vi "FFT Testing.vi"() -> ()   [LabVIEW 2019]
uses:
  <vilib>/express/express analysis/Spectral/Block/exnSpectralBlock spectral measurements peak poly.vi
  <vilib>/express/express analysis/Spectral/Block/exnSpectralBlock spectral measurements peak DDT.vi
  <vilib>/express/express analysis/Spectral/XNode/ExpressSpectralMeasurementsBlockNode.xnode
panel:
  out "Freq Max":dbl
  out "Amp":dbl
  out "data":dynamicdata(graph)
  out "Waveform Graph 2":dynamicdata(graph)
  in  "stop (F)":bool
  out "Waveform Graph":dynamicdata(graph)
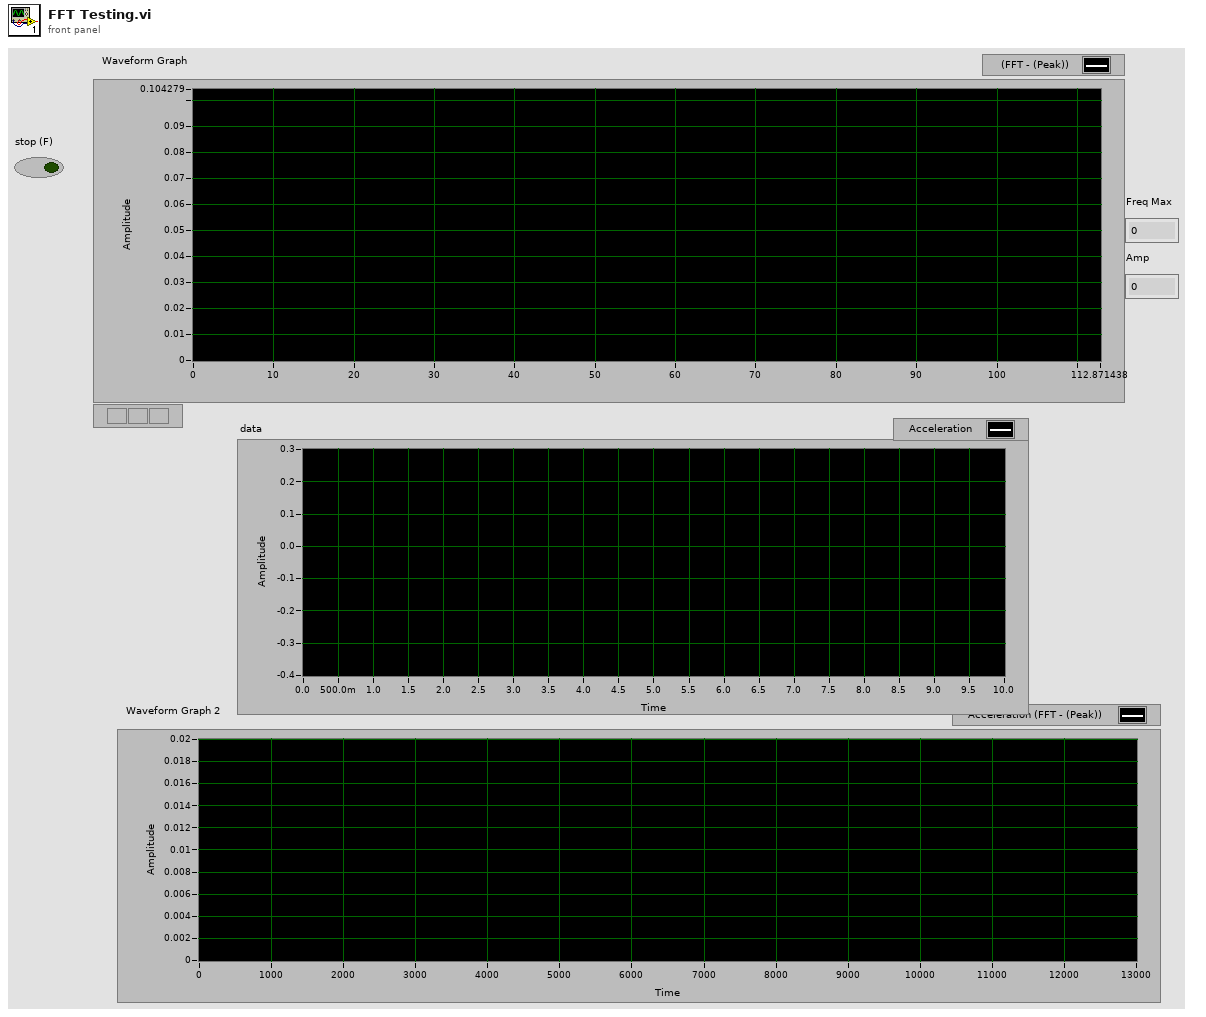
[diagram p1: front panel]
types:
  T1 = cluster{"averaging mode":u16, "weighting mode":u16, "number of averages":u32}
  T2 = cluster{"dB On (F)":bool, "unwrap phase (F)":bool, "convert to degree (F)":bool}
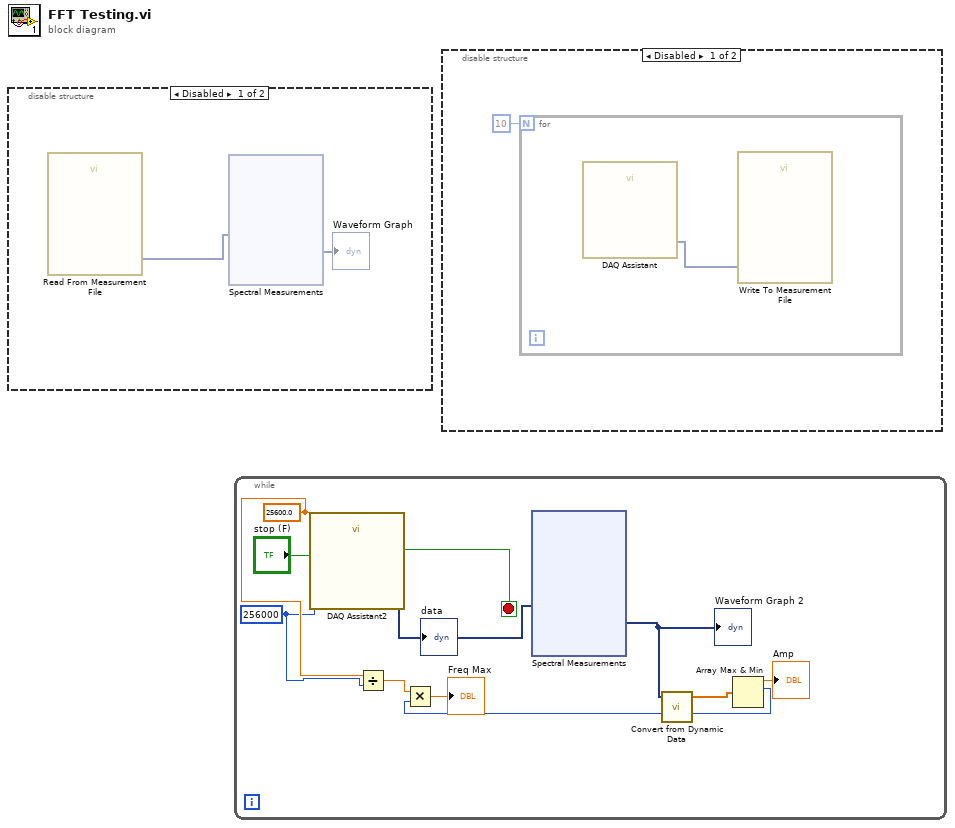
[diagram p0: block diagram]
diagram:
  n1 = disable-structure shown="Disabled" {
    frame Disabled {
      n2 = call "Read From Measurement File"() -> ("Signals"=w1:dynamicdata)  [unwired: 6 in, 5 out]
      n3 = xnode "Spectral Measurements"("Signals"=w1) -> ("FFT - (Peak)"=→"Waveform Graph":dynamicdata)  [unwired: 1 in, 2 out]
    }
    frame Enabled {
    }
  }
  n4 = while {
    stop <- w22 stop-if-true
    w17 = 256000 ("number of samples")
    w18 = 25600.0 ("rate")
    n5 = call "DAQ Assistant2"("rate"=w18, "number of samples"=w17, "stop (F)"="stop (F)") -> ("data"=w21:dynamicdata, "stopped"=w22:bool)  [unwired: 13 in, 2 out]
    "data" <- w21
    n6 = Divide(x=w18, y=w17) -> (x/y=w16:dbl)
    n7 = xnode "Spectral Measurements"("Signals"=w21) -> ("FFT - (Peak)"=w20:dynamicdata)  [unwired: 1 in, 2 out]
    "Waveform Graph 2" <- w20
    n8 = call "Convert from Dynamic Data"("Dynamic Data Type"=w20) -> ("Array"=w19:dbl[])  [unwired: 3 in]
    n9 = Array Max & Min(array=w19) -> (max value=→"Amp":dbl, max index (indices)=w15:i32)  [unwired: 2 out]
    n10 = Multiply(x=w16, y=w15) -> (x*y=→"Freq Max":dbl)
  }
  n11 = disable-structure shown="Disabled" {
    frame Disabled {
      n12 = for {
        N: 10 -> [_]
        n13 = call "DAQ Assistant"() -> ("data"=w35:dynamicdata)  [unwired: 17 in, 2 out]
        n14 = call "Write To Measurement File"("Signals"=w35) -> ()  [unwired: 16 in, 3 out]
      }
    }
    frame Enabled {
    }
  }
